vi "Get QueueByPriorityNumber.vi"(8 "error in (no error)":errorcluster, 10 "Priority Number":i32, 11 "PriorityQueue in":refnum<class "PriorityQueue.lvclass">) -> (0 "error out":errorcluster, 2 "Internal Queue":refnum<queue>, 3 "PriorityQueue out":refnum<class "PriorityQueue.lvclass">)   [LabVIEW 2019, in "PriorityQueue.lvclass"]
doc: "PRIVATE METHOD - DO NOT EXPOSE EXTERNALLY\n\nRetrieves the queue representing the correct priority number. This vi implements the default behavior for situations when the specified priority number is out of bounds."
uses:
  PriorityQueue.lvclass
  PriorityQueue.lvclass/PriorityQueue.ctl
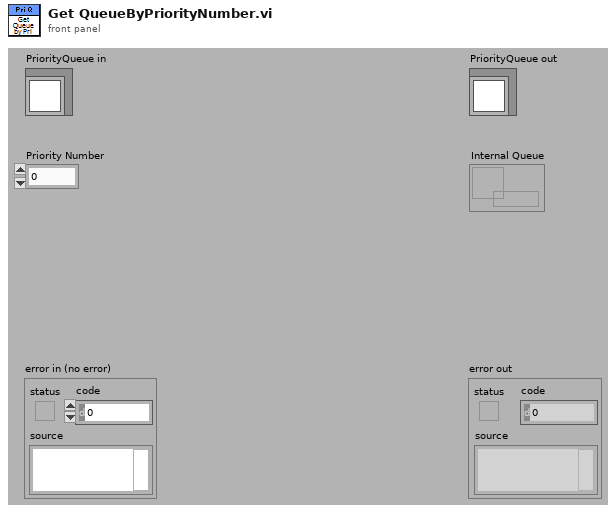
[diagram p1: front panel]
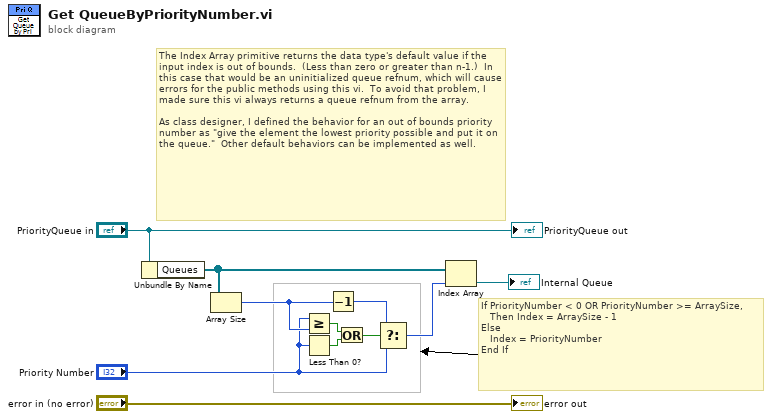
[diagram p0: block diagram]
diagram:
  # "The Index Array primitive returns the data type's default value if the input index is out of bounds.  (Less than zero or greater than n-1.)  In this case that would be an uninitialized queue refnum, which will cause errors for the public methods using this vi.  To avoid that problem, I made sure this vi always returns a queue refnum from the array.\n\nAs class designer, I defined the behavior for an out of bounds priority number as \"give the element the lowest priority possible and put it on the queue.\"  Other default behaviors can be implemented as well."
  # "If PriorityNumber < 0 OR PriorityNumber >= ArraySize,\n   Then Index = ArraySize - 1\nElse\n   Index = PriorityNumber\nEnd If"
  n1 = Unbundle By Name("PriorityQueue in") -> ("Queues"=w10:refnum<queue>[])
  n2 = Array Size(array=w10) -> (size(s)=w6:i32)
  n3 = Greater Or Equal?(x="Priority Number", y=w6) -> (x >= y?=w9:bool)
  n4 = Less Than 0?(x="Priority Number") -> (x < 0?=w8:bool)
  n5 = Decrement(x=w6) -> (x-1=w1:i32)
  n6 = Or(x=w9, y=w8) -> (x .or. y?=w7:bool)
  n7 = Select(t=w1, s=w7, f="Priority Number") -> (s? t:f=w4:i32)
  n8 = Index Array(array=w10, index=w4) -> (element=→"Internal Queue":refnum<queue>)
  "error out" <- "error in (no error)"
  "PriorityQueue out" <- "PriorityQueue in"
